vi "Username_Password.vi"() -> ()   [LabVIEW 2024]
panel:
  out "x = y?":bool
  in  "Password":string
  in  "Username":string
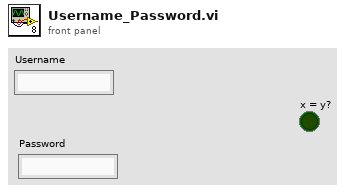
[diagram p1: front panel]
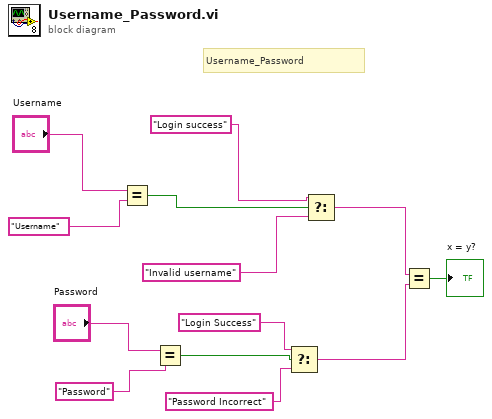
[diagram p0: block diagram]
diagram:
  # "Username_Password"
  n1 = Equal?(x="Username", y="Username" ("true string")) -> (x = y?=w11:bool)
  n2 = Equal?(x="Password", y="Password" ("true string")) -> (x = y?=w10:bool)
  n3 = Select(t="Login Success" ("true string"), s=w10, f="Password Incorrect" ("true string")) -> (s? t:f=w3:string)
  n4 = Select(t="Login success" ("true string"), s=w11, f="Invalid username" ("true string")) -> (s? t:f=w1:string)
  n5 = Equal?(x=w1, y=w3) -> (x = y?=→"x = y?":bool)
